vi "Kyle's Move to Wavelength.vi"(7 "Mono System # (0)":T1, 8 "error in (no error)":errorcluster, 10 "Target Wavelength\nGPIB":dbl[unit], 11 "VISA resource name":refnum<visa-resource-name>) -> (0 "error out":errorcluster, 3 "VISA resource name out":refnum<visa-resource-name>)   [LabVIEW 2009, in "JY-SPEX-TRIAX.lvlib"]
doc: "Moves the spectrometer's grating to a specific wavelength according to the base grating (1200 grooves/mm).\n\n<B>Note: only works with TRIAX series monochromators.</B>"
uses:
  JY-SPEX-TRIAX.lvlib
  controls.llb/Monochromator System Number.ctl
  Spectrometer Config.vi
  Synapse CCD/Control Panel.vi
  Control Panel.vi
  Synapse CCD/Synapse CCD.lvclass
  Spectrometer Triax 550.lvclass
panel:
  in  "Read":bool
  out "Last wavelength":dbl[unit]
  in  "Target Wavelength\nActiveX":dbl[unit]
  out "Wavelength ActiveX":dbl[unit]
  in  "ActiveX":bool
  in  "GPIB":bool
  in  "stop":bool
  out "True if correcting\nfor Grating C":bool
  out "Wavelength GPIB":dbl[unit]
  out "Backlash":dbl[unit]
  out "Distance":dbl[unit]
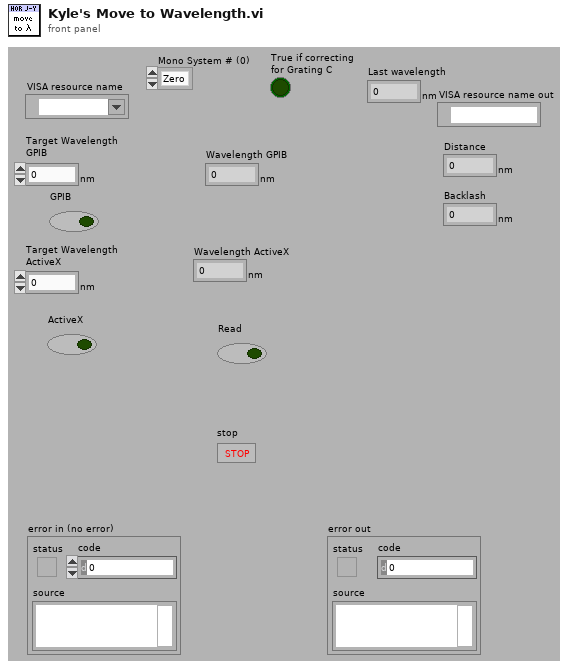
[diagram p1: front panel]
types:
  T1 = typedef "JY-SPEX-TRIAX.lvlib/Monochromator System Number.ctl" = enum16{"Zero", "One"}
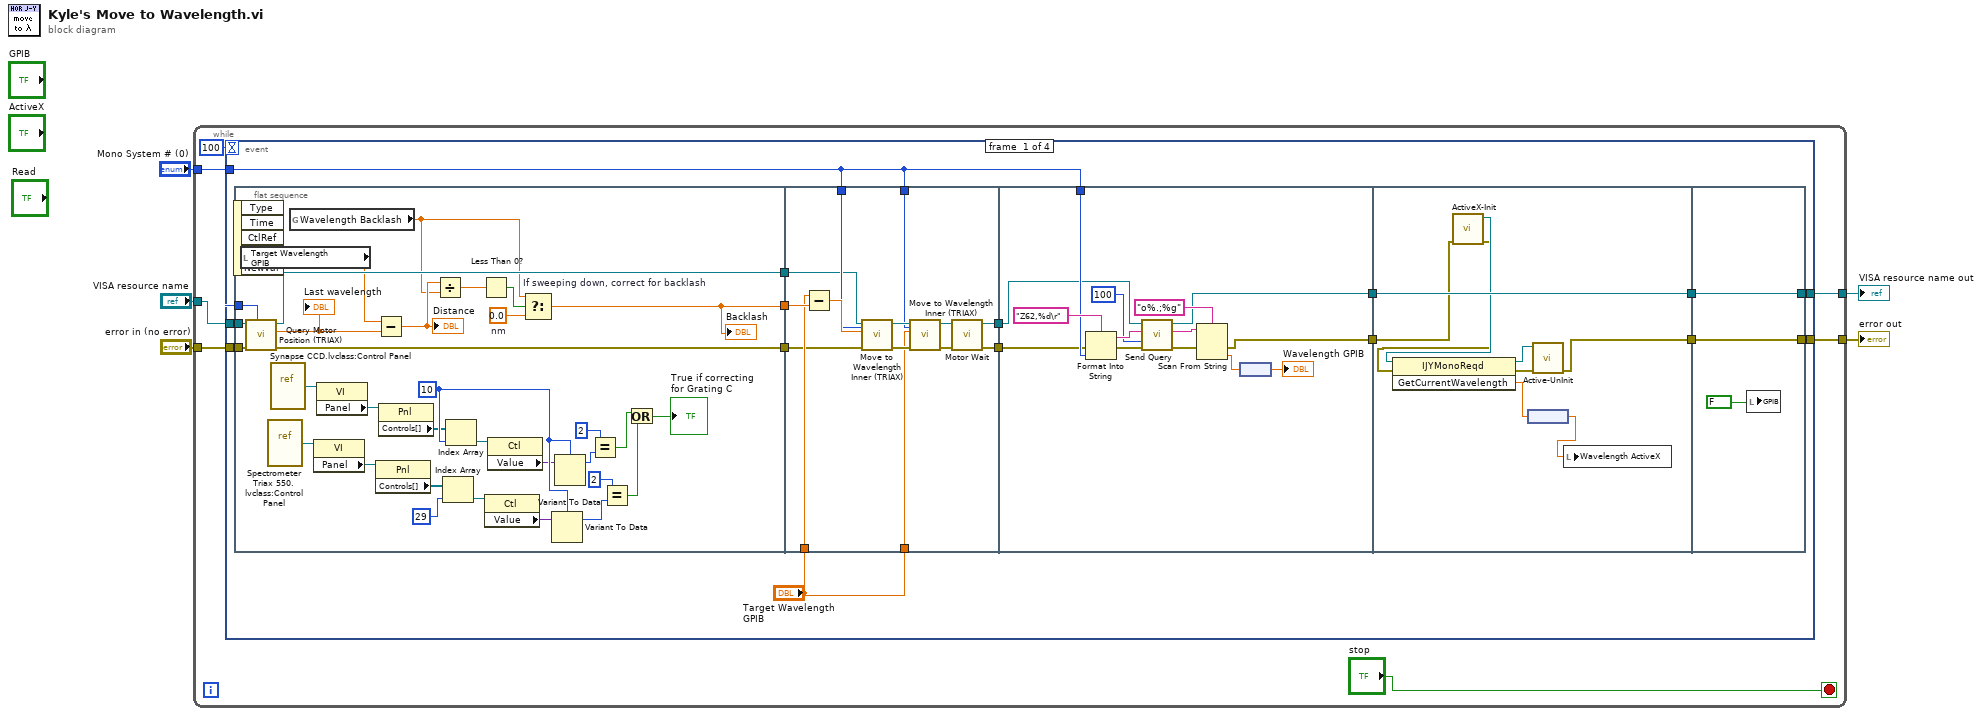
[diagram p0: block diagram]
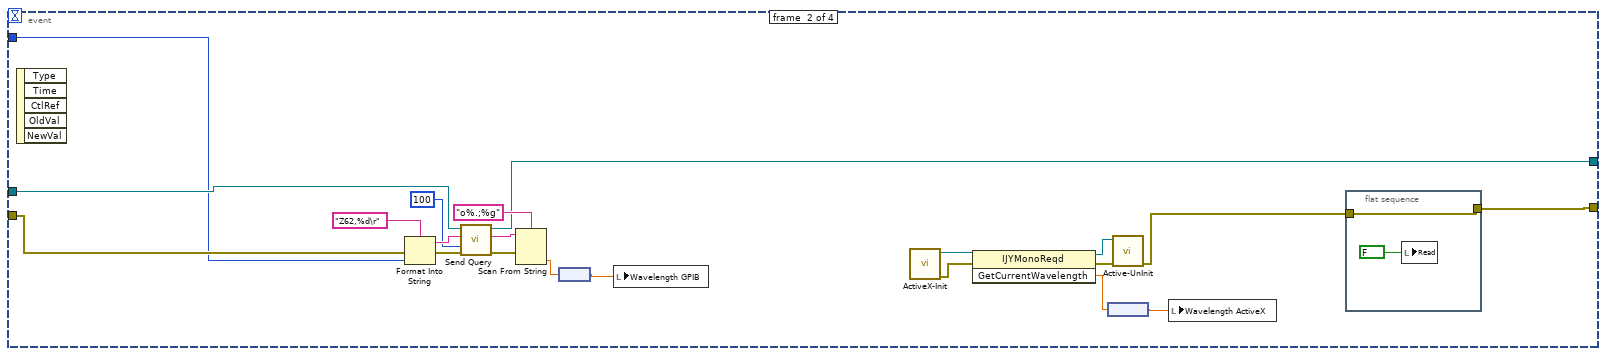
[diagram p2: hidden frame]
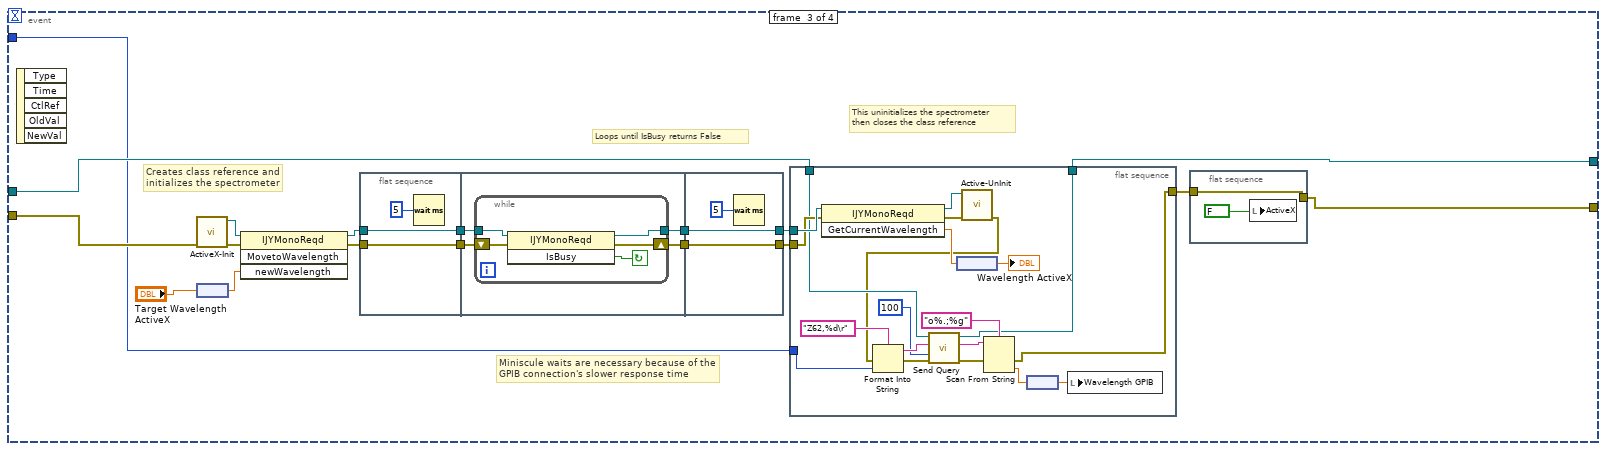
[diagram p3: hidden frame]
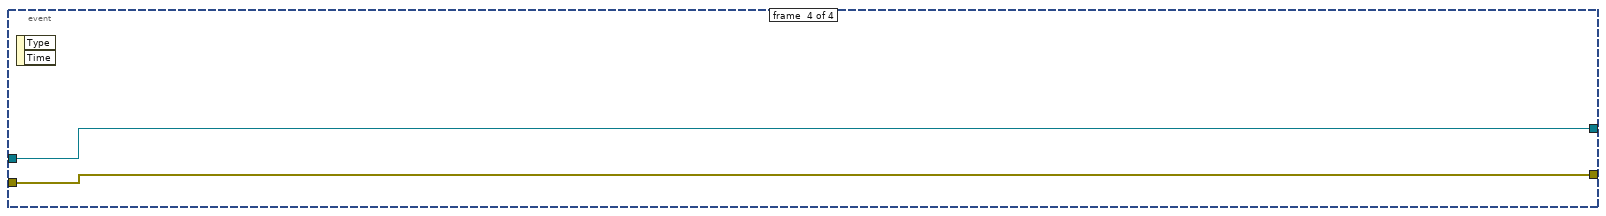
[diagram p4: hidden frame]
diagram:
  n1 = while {
    tunnel: "VISA resource name" -> [w12]
    tunnel: "error in (no error)" -> [w11]
    tunnel: "Mono System # (0)" -> [w10]
    tunnel: [w9] -> w2
    tunnel: [w8] -> w1
    stop <- "stop" stop-if-true
    n2 = event shown="[1] \"Read\": Value Change" {
      selector: _ -> [_ _ _ _]
      dyn-events: _ -> [_ _ _ _]
      timeout: 100 -> [_ _ _ _]
      tunnel: w12 -> [w22 w106 w125 w179]
      tunnel: w11 -> [w21 w105 w130 w178]
      tunnel: w10 -> [w20 w104 w123 _]
      tunnel: [w19 w102 w124 w179] -> w9
      tunnel: [w18 w101 w126 w178] -> w8
      event #0 {
        n3 = event-data() -> ()  [unwired: 1 in, 5 out]
        n4 = flat-sequence {
          tunnel: w22 -> [w59]
          tunnel: w21 -> [w57]
          tunnel: w20 -> [w53]
          tunnel: [w58] -> w27
          tunnel: [w56] -> w26
          tunnel: [w47] -> w25
          tunnel: w27 -> [w63]
          tunnel: w26 -> [w62]
          tunnel: w25 -> [w68]
          tunnel: "Target Wavelength\nGPIB" -> [w67]
          tunnel: "Target Wavelength\nGPIB" -> [w64]
          tunnel: w20 -> [w66]
          tunnel: w20 -> [w65]
          tunnel: [w61] -> w24
          tunnel: [w60] -> w23
          tunnel: w20 -> [w78]
          tunnel: w24 -> [w77]
          tunnel: w23 -> [w76]
          tunnel: [w75] -> w16
          tunnel: [w74] -> w14
          tunnel: w16 -> [w96]
          tunnel: [w96] -> w15
          tunnel: w14 -> [w95]
          tunnel: [w88] -> w13
          tunnel: [w98] -> w18
          tunnel: [w99] -> w19
          tunnel: w15 -> [w99]
          tunnel: w13 -> [w98]
          frame #0 {
            w38 = 10
            w48 = dbl[unit] 0.0  # nm
            n5 = local read "Target Wavelength\nGPIB"() -> (w55:dbl[unit])
            n6 = call "Query Motor Position (TRIAX).vi"("Mono System # (0)"=w53, "error in (no error)"=w57, "VISA resource name"=w59) -> ("error out"=w56:errorcluster, "wavelength"=w54:dbl[unit], "VISA resource name out"=w58:refnum<visa-resource-name>)  [unwired: 6 out]
            "Last wavelength" <- w54
            n7 = vi-ref "Spectrometer Triax 550.lvclass:Control Panel.vi"() -> (w33:refnum<vi>)
            n8 = vi-ref "Synapse CCD.lvclass:Control Panel.vi"() -> (w28:refnum<vi>)
            n9 = global read "Spectrometer Config.vi" "Wavelength Backlash"() -> (w49:dbl[unit])
            n10 = property class="VI"(reference=w33) -> ("Panel"=w34:refnum<vi>)  [unwired: 1 in, 2 out]
            n11 = property class="VI"(reference=w28) -> ("Panel"=w29:refnum<vi>)  [unwired: 1 in, 2 out]
            n12 = Subtract(x=w55, y=w54) -> (x-y=w50:dbl[unit])
            "Distance" <- w50
            n13 = property class="Pnl"(reference=w34) -> ("Controls[]"=w35:refnum<vi>[])  [unwired: 1 in, 2 out]
            n14 = property class="Pnl"(reference=w29) -> ("Controls[]"=w30:refnum<vi>[])  [unwired: 1 in, 2 out]
            n15 = Divide(x=w50, y=w49) -> (x/y=w51:dbl)
            n16 = Index Array(array=w35, index=29) -> (element=w36:refnum<vi>)
            n17 = Index Array(array=w30, index=w38) -> (element=w31:refnum<vi>)
            n18 = Less Than 0?(x=w51) -> (x < 0?=w52:bool)
            n19 = property class="Ctl"(reference=w36) -> ("Value"=w37:variant)  [unwired: 1 in, 2 out]
            n20 = property class="Ctl"(reference=w31) -> ("Value"=w32:variant)  [unwired: 1 in, 2 out]
            n21 = Select "If sweeping down, correct for backlash"(t=w49, s=w52, f=w48) -> (s? t:f=w47:dbl[unit])
            "Backlash" <- w47
            n22 = Variant To Data(Variant=w37, type=w38) -> (data=w42:i32)  [unwired: 1 in, 1 out]
            n23 = Variant To Data(Variant=w32, type=w38) -> (data=w40:i32)  [unwired: 1 in, 1 out]
            n24 = Equal?(x=2, y=w40) -> (x = y?=w43:bool)
            n25 = Equal?(x=2, y=w42) -> (x = y?=w44:bool)
            n26 = Or(x=w43, y=w44) -> (x .or. y?=→"True if correcting\nfor Grating C":bool)
          }
          frame #1 {
            n27 = Subtract(x=w67, y=w68) -> (x-y=w71:dbl[unit])
            n28 = call "Move to Wavelength Inner (TRIAX).vi"("Mono System # (0)"=w66, "error in (no error)"=w62, "wavelength"=w71, "VISA resource name"=w63) -> ("error out"=w70:errorcluster, "VISA resource name out"=w69:refnum<visa-resource-name>)  [unwired: 6 out]
            n29 = call "Move to Wavelength Inner (TRIAX).vi"("Mono System # (0)"=w65, "error in (no error)"=w70, "wavelength"=w64, "VISA resource name"=w69) -> ("error out"=w73:errorcluster, "VISA resource name out"=w72:refnum<visa-resource-name>)  [unwired: 6 out]
            n30 = call "Motor Wait.vi"("error in"=w73, "VISA resource name in"=w72) -> ("error out"=w61:errorcluster, "VISA resource name out"=w60:refnum<visa-resource-name>)  [unwired: 8 out]
          }
          frame #2 {
            n31 = Format Into String(format string="Z62,%d\r", error in=w77, w78) -> (resulting string=w85:string, error out=w86:errorcluster)  [unwired: 1 in]
            n32 = call "Send Query.vi"("error in (no error)"=w86, "byte count"=u32 100, "write buffer"=w85, "VISA resource name"=w76) -> ("error out"=w82:errorcluster, "read buffer"=w80:string, "VISA resource name out"=w75:refnum<visa-resource-name>)  [unwired: 5 out]
            n33 = Scan From String(format string="o%.;%g", input string=w80, error in=w82) -> (error out=w74:errorcluster, output 1=w87:dbl)  [unwired: 1 in, 3 out]
            n34 = node(w87) -> (→"Wavelength GPIB":dbl[unit])
          }
          frame #3 {
            n35 = call "ActiveX-Init.vi"("error in (no error)"=w95) -> ("error out"=w90:errorcluster, "TRIAX Out"=w91:refnum<k7>)  [unwired: 9 in]
            n36 = invoke class="IJYMonoReqd" method="GetCurrentWavelength"(reference=w91, error in=w90) -> (reference out=w94:refnum<k7>, error out=w93:errorcluster, "GetCurrentWavelength"=w92:dbl)  [unwired: 1 in]
            n37 = node(w92) -> (w89:dbl[unit])
            n38 = call "Active-UnInit.vi"("error in (no error)"=w93, "TRIAX In"=w94) -> ("error out"=w88:errorcluster)  [unwired: 9 in]
            n39 = local write "Wavelength ActiveX"(w89) -> ()
          }
          frame #4 {
            n40 = local write "GPIB"(FALSE) -> ()
          }
        }
      }
      event #1 {
        n41 = event-data() -> ()  [unwired: 1 in, 5 out]
        n42 = Format Into String(format string="Z62,%d\r", error in=w105, w104) -> (resulting string=w112:string, error out=w113:errorcluster)  [unwired: 1 in]
        n43 = call "Send Query.vi"("error in (no error)"=w113, "byte count"=u32 100, "write buffer"=w112, "VISA resource name"=w106) -> ("error out"=w110:errorcluster, "read buffer"=w108:string, "VISA resource name out"=w102:refnum<visa-resource-name>)  [unwired: 5 out]
        n44 = Scan From String(format string="o%.;%g", input string=w108, error in=w110) -> (output 1=w114:dbl)  [unwired: 1 in, 4 out]
        n45 = node(w114) -> (w103:dbl[unit])
        n46 = local write "Wavelength GPIB"(w103) -> ()
        n47 = call "ActiveX-Init.vi"() -> ("error out"=w116:errorcluster, "TRIAX Out"=w115:refnum<k7>)  [unwired: 10 in]
        n48 = invoke class="IJYMonoReqd" method="GetCurrentWavelength"(reference=w115, error in=w116) -> (reference out=w120:refnum<k7>, error out=w119:errorcluster, "GetCurrentWavelength"=w118:dbl)  [unwired: 1 in]
        n49 = node(w118) -> (w117:dbl[unit])
        n50 = call "Active-UnInit.vi"("error in (no error)"=w119, "TRIAX In"=w120) -> ("error out"=w100:errorcluster)  [unwired: 9 in]
        n51 = local write "Wavelength ActiveX"(w117) -> ()
        n52 = flat-sequence {
          tunnel: [w122] -> w101
          tunnel: w100 -> [w122]
          frame #0 {
            n53 = local write "Read"(FALSE) -> ()
          }
        }
      }
      event #2 {
        # "This uninitializes the spectrometer\nthen closes the class reference"
        # "Creates class reference and\ninitializes the spectrometer"
        # "Miniscule waits are necessary because of the \nGPIB connection's slower response time"
        # "Loops until IsBusy returns False"
        n54 = event-data() -> ()  [unwired: 1 in, 5 out]
        n55 = call "ActiveX-Init.vi"("error in (no error)"=w130) -> ("error out"=w135:errorcluster, "TRIAX Out"=w136:refnum<k7>)  [unwired: 9 in]
        n56 = node("Target Wavelength\nActiveX") -> (w129:dbl)
        n57 = invoke class="IJYMonoReqd" method="MovetoWavelength"(reference=w136, error in=w135, "newWavelength"=w129) -> (reference out=w132:refnum<k7>, error out=w131:errorcluster)  [unwired: 1 in, 2 out]
        n58 = flat-sequence {
          tunnel: w132 -> [w164]
          tunnel: [w164] -> w140
          tunnel: w131 -> [w163]
          tunnel: [w163] -> w139
          tunnel: [w167] -> w138
          tunnel: w140 -> [w169]
          tunnel: w139 -> [w168]
          tunnel: [w166] -> w137
          tunnel: [w176] -> w134
          tunnel: [w175] -> w133
          tunnel: w138 -> [w176]
          tunnel: w137 -> [w175]
          frame #0 {
            n59 = Wait (ms)(milliseconds to wait=u32 5) -> ()  [unwired: 1 out]
          }
          frame #1 {
            n60 = while {
              tunnel: w169 -> [w174]
              shift-right: [w170] -> w166
              shift-left: w168 -> [w173]
              tunnel: [w171] -> w167
              stop <- w172 continue-if-true
              n61 = invoke class="IJYMonoReqd" method="IsBusy"(reference=w174, error in=w173) -> (reference out=w171:refnum<k7>, error out=w170:errorcluster, "IsBusy"=w172:bool)  [unwired: 1 in]
            }
          }
          frame #2 {
            n62 = Wait (ms)(milliseconds to wait=u32 5) -> ()  [unwired: 1 out]
          }
        }
        n63 = flat-sequence {
          tunnel: w134 -> [w156]
          tunnel: w133 -> [w147]
          tunnel: [w146] -> w127
          tunnel: w125 -> [w145]
          tunnel: [w144] -> w124
          tunnel: w123 -> [w142]
          frame #0 {
            n64 = invoke class="IJYMonoReqd" method="GetCurrentWavelength"(reference=w156, error in=w147) -> (reference out=w160:refnum<k7>, error out=w159:errorcluster, "GetCurrentWavelength"=w158:dbl)  [unwired: 1 in]
            n65 = node(w158) -> (→"Wavelength ActiveX":dbl[unit])
            n66 = call "Active-UnInit.vi"("error in (no error)"=w159, "TRIAX In"=w160) -> ("error out"=w143:errorcluster)  [unwired: 9 in]
            n67 = Format Into String(format string="Z62,%d\r", error in=w143, w142) -> (resulting string=w153:string, error out=w154:errorcluster)  [unwired: 1 in]
            n68 = call "Send Query.vi"("error in (no error)"=w154, "byte count"=u32 100, "write buffer"=w153, "VISA resource name"=w145) -> ("error out"=w151:errorcluster, "read buffer"=w149:string, "VISA resource name out"=w144:refnum<visa-resource-name>)  [unwired: 5 out]
            n69 = Scan From String(format string="o%.;%g", input string=w149, error in=w151) -> (error out=w146:errorcluster, output 1=w155:dbl)  [unwired: 1 in, 3 out]
            n70 = node(w155) -> (w141:dbl[unit])
            n71 = local write "Wavelength GPIB"(w141) -> ()
          }
        }
        n72 = flat-sequence {
          tunnel: [w161] -> w126
          tunnel: w127 -> [w161]
          frame #0 {
            n73 = local write "ActiveX"(FALSE) -> ()
          }
        }
      }
      event #3 {
        n74 = event-data() -> ()  [unwired: 1 in, 2 out]
      }
    }
  }
  "error out" <- w1
  "VISA resource name out" <- w2
